vi "Go.vi"(8 "Timing Data (Go Down and Dispense)":T1(array[cluster]), 9 "Timing Values":dbl[](array[numeric]), 10 "Control In":T2={"I-O.lvclass"=refnum, "Motion.lvclass"=refnum, "Dispenser.lvclass"=refnum}, 11 "CAD Dispense in":refnum<class "CAD Dispense.lvclass">) -> (2 "Control Out":T2, 3 "CAD Dispense Out":refnum<class "CAD Dispense.lvclass">)   [LabVIEW 2016, in "CAD Dispense.lvclass"]
uses:
  CAD Dispense.lvclass
  Controller/Controllers.ctl
  Controller/I-O/I-O.lvclass
  Controller/Motion/A3200/A3200.lvclass
  Controller/Dispenser/Dispenser.lvclass
  Controller/Motion/Motion.lvclass
  CAD Dispense.lvclass/CAD Dispense.ctl
  Controller/Controller.lvclass
panel:
  out "Numeric":i32
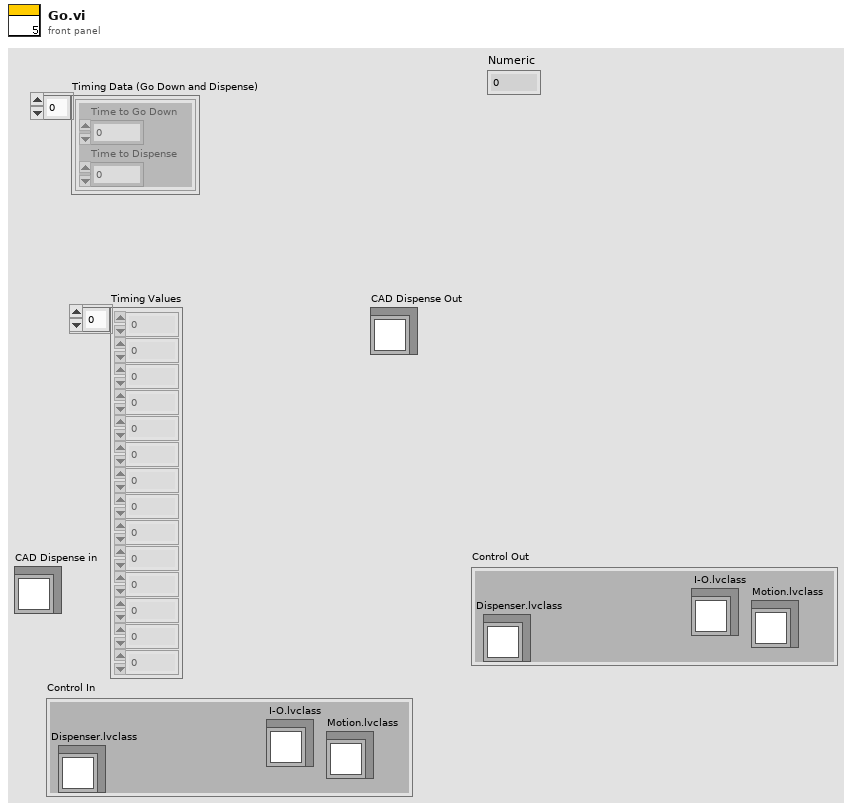
[diagram p1: front panel]
types:
  T1 = cluster{"Time to Go Down":dbl, "Time to Dispense":dbl}[]
  T2 = typedef "Controller.lvclass/Controllers.ctl" = cluster{"I-O.lvclass":refnum<class "I-O.lvclass">, "Motion.lvclass":refnum<class "Motion.lvclass">, "Dispenser.lvclass":refnum<class "Dispenser.lvclass">}
  T3 = cluster{"Motion":dbl[][], "Center":dbl[], "Circle?":bool, "CW/CCW":dbl}[]
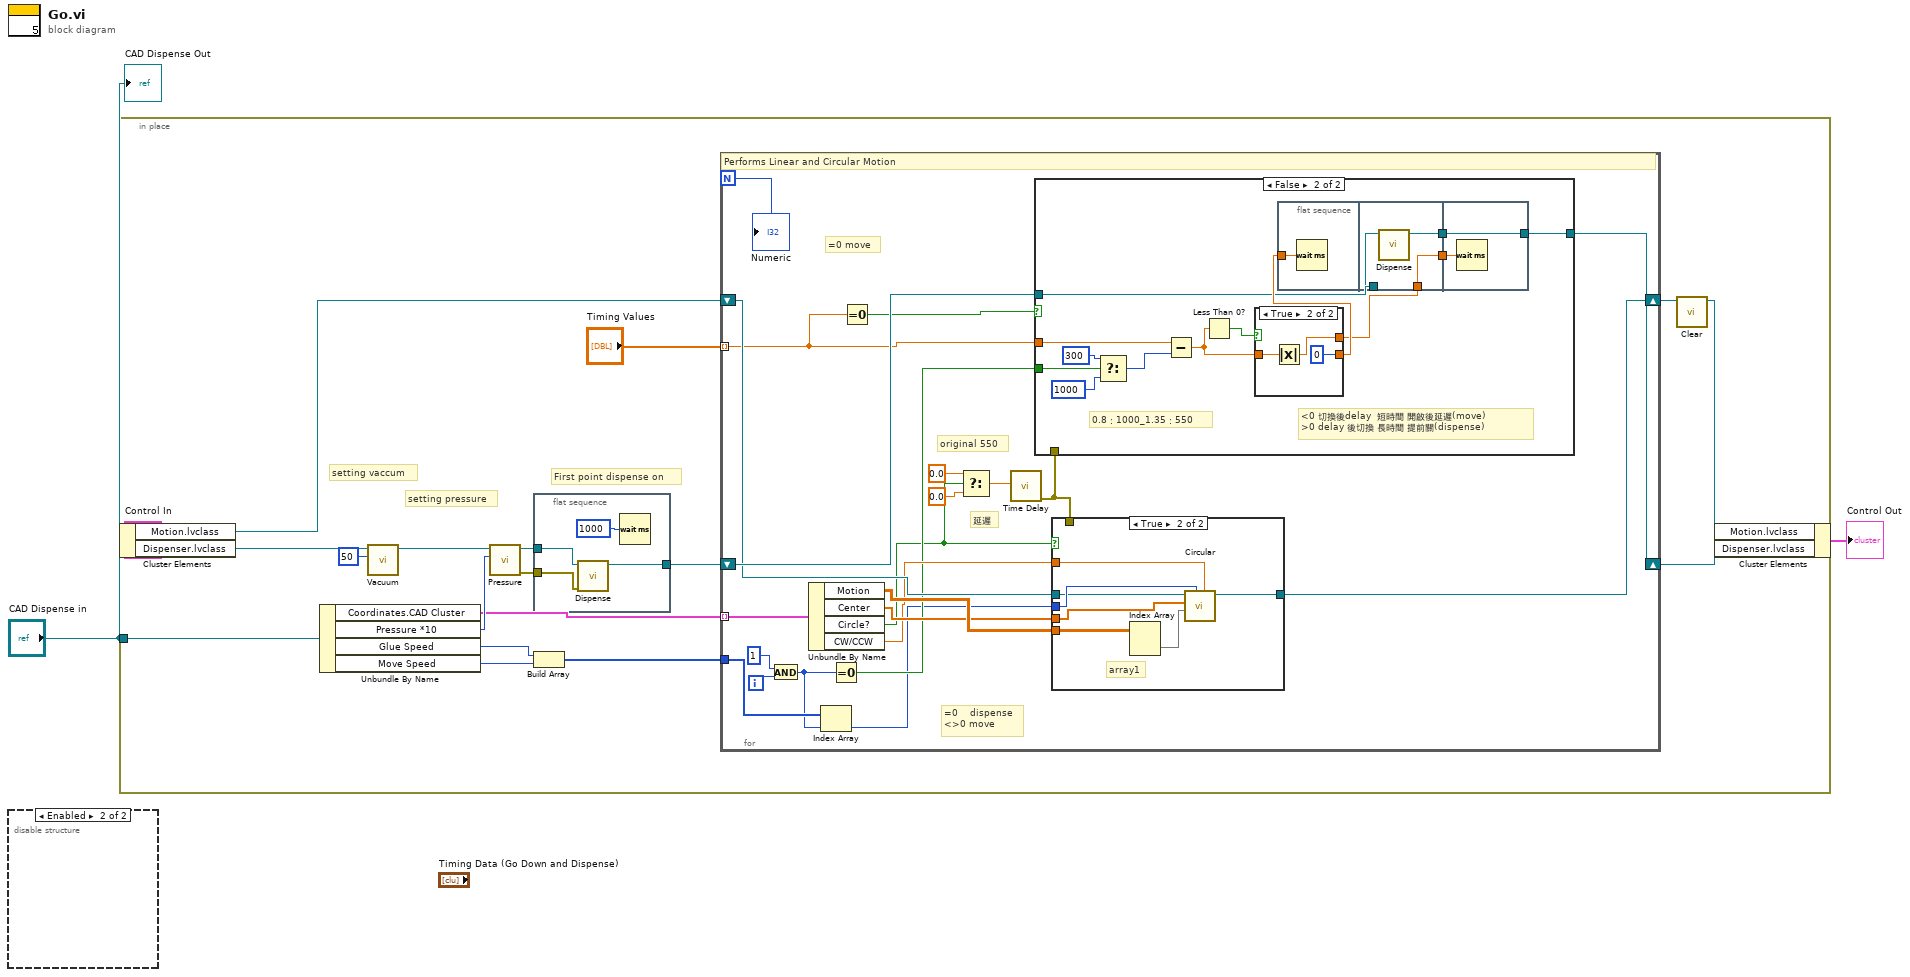
[diagram p0: block diagram]
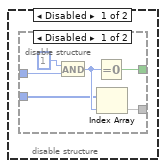
[diagram p2: hidden frame]
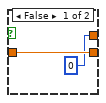
[diagram p5: hidden frame]
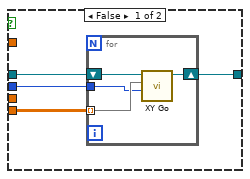
[diagram p6: hidden frame]
diagram:
  n1 = disable-structure shown="Enabled" {
    frame Disabled {
      n2 = disable-structure shown="Disabled" {
        disable-tunnel: [w8 _] -> _
        disable-tunnel: _ -> [w7 _]
        disable-tunnel: [w5 _] -> _
        disable-tunnel: _ -> [w4 _]
        frame Disabled {
          n3 = And(x=1, y=w7) -> (x .and. y?=w6:i32)
          n4 = Equal To 0?(x=w6) -> (x = 0?=w5:bool)
          n5 = Index Array(array=w4, index=w6) -> (element=w8)
        }
        frame Enabled {
        }
      }
    }
    frame Enabled {
    }
  }
  n6 = in-place {
    in-place-border: "CAD Dispense in" -> [w25]
    # "setting pressure"
    # "setting vaccum"
    # "First point dispense on"
    n7 = in-place-cluster #1("Control In") -> ("Motion.lvclass"=w19:refnum<class "Motion.lvclass">, "Dispenser.lvclass"=w12:refnum<class "Dispenser.lvclass">)
    n8 = Unbundle By Name(w25) -> ("Coordinates.CAD Cluster"=w13:T3, "Pressure *10"=w16:i64, "Glue Speed"=w23:i32, "Move Speed"=w22:i32)
    n9 = call-dynamic "Vacuum.vi"("Vacuum Setting (0000)"=i64 50, "Dispenser in"=w12) -> ("Dispenser out"=w11:refnum<class "Dispenser.lvclass">)  [unwired: 8 in, 1 out]
    n10 = call-dynamic "Pressure.vi"("Pressure"=w16, "Dispenser in"=w11) -> ("error out"=w15:errorcluster, "Dispenser out"=w14:refnum<class "Dispenser.lvclass">)  [unwired: 8 in]
    n11 = flat-sequence {
      tunnel: [w28] -> w24
      tunnel: w15 -> [w27]
      tunnel: w14 -> [w29]
      frame #0 {
        n12 = call-dynamic "Dispense.vi"("error in (no error)"=w27, "Dispenser in"=w29) -> ("Dispenser out"=w28:refnum<class "Dispenser.lvclass">)  [unwired: 8 in, 1 out]
        n13 = Wait (ms)(milliseconds to wait=u32 1000) -> ()  [unwired: 1 out]
      }
    }
    n14 = Build Array(w23, w22) -> (w21:i32[])
    n15 = for {
      N -> [w31]
      tunnel: w13 -> [w51] mode=indexing
      tunnel: "Timing Values" -> [w38] mode=indexing
      tunnel: w21 -> [w44]
      shift-right: [w46] -> w26
      shift-left: w24 -> [w52]
      shift-right: [w45] -> w18
      shift-left: w19 -> [w48]
      i -> [w43]
      # "=0 move"
      # "=0    dispense\n<>0 move"
      # "延遲"
      # "original 550"
      # "Performs Linear and Circular Motion"
      n16 = And(x=1, y=w43) -> (x .and. y?=w41:i32)
      n17 = Unbundle By Name(w51) -> ("Motion"=w50:dbl[][], "Center"=w49:dbl[], "Circle?"=w36:bool, "CW/CCW"=w47:dbl)
      n18 = Index Array(array=w44, index=w41) -> (element=w39:i32)
      n19 = Equal To 0?(x=w41) -> (x = 0?=w40:bool)
      n20 = Equal To 0?(x=w38) -> (x = 0?=w37:bool)
      n21 = Select(t=0.0, s=w36, f=0.0) -> (s? t:f=w33:dbl)
      n22 = call "Time Delay"("Delay Time (s)"=w33) -> ("error out"=w32:errorcluster)  [unwired: 10 in]
      n23 = case shown="False" w37 {
        tunnel: w52 -> [w53 w61]
        tunnel: w38 -> [_ w58]
        tunnel: [w53 w57] -> w46
        tunnel: w40 -> [_ w56]
        tunnel: w32 -> [_ _]
        frame True {
        }
        frame False {
          # "<0 切換後delay  短時間 開啟後延遲(move)\n>0 delay 後切換 長時間 提前關(dispense)"
          # "0.8：1000_1.35：550"
          n24 = Select(t=300, s=w56, f=1000) -> (s? t:f=w60:i32)
          n25 = Subtract(x=w58, y=w60) -> (x-y=w59:dbl)
          n26 = Less Than 0?(x=w59) -> (x < 0?=w64:bool)
          n27 = case shown="True" w64 {
            tunnel: [w74 u32 0 ("milliseconds to wait")] -> w63
            tunnel: w59 -> [w74 w77]
            tunnel: [u32 0 ("milliseconds to wait") w76] -> w62
            frame False {
            }
            frame True {
              n28 = Absolute Value(x=w77) -> (abs(x)=w76:dbl)
            }
          }
          n29 = flat-sequence {
            tunnel: w63 -> [w67]
            tunnel: w61 -> [w69]
            tunnel: [w70] -> w66
            tunnel: w62 -> [w70]
            tunnel: [w68] -> w65
            tunnel: w66 -> [w72]
            tunnel: w65 -> [w71]
            tunnel: [w71] -> w57
            frame #0 {
              n30 = Wait (ms)(milliseconds to wait=w67) -> ()  [unwired: 1 out]
            }
            frame #1 {
              n31 = call-dynamic "Dispense.vi"("Dispenser in"=w69) -> ("Dispenser out"=w68:refnum<class "Dispenser.lvclass">)  [unwired: 9 in, 1 out]
            }
            frame #2 {
              n32 = Wait (ms)(milliseconds to wait=w72) -> ()  [unwired: 1 out]
            }
          }
        }
      }
      n33 = case shown="True" w36 {
        tunnel: [w78 w86] -> w45
        tunnel: w47 -> [_ w89]
        tunnel: w50 -> [w80 w92]
        tunnel: w49 -> [_ w91]
        tunnel: w48 -> [w81 w87]
        tunnel: w39 -> [w79 w88]
        tunnel: w32 -> [_ _]
        frame False {
          n34 = for {
            tunnel: w80 -> [w84] mode=indexing
            shift-right: [w85] -> w78
            shift-left: w81 -> [w82]
            tunnel: w79 -> [w83]
            n35 = call-dynamic "XY Go.vi"("Speed"=w83, "XY"=w84, "Motion in"=w82) -> ("Motion out"=w85:refnum<class "Motion.lvclass">)  [unwired: 7 in, 1 out]
          }
        }
        frame True {
          # "array1"
          n36 = Index Array(array=w92) -> (element=w90:dbl[])  [unwired: 2 in]
          n37 = call-dynamic "Circular.vi"("Direction"=w89, "Speed"=w88, "XY End"=w90, "XY Center"=w91, "Motion in"=w87) -> ("Motion out"=w86:refnum<class "Motion.lvclass">)  [unwired: 5 in, 1 out]
        }
      }
      "Numeric" <- w31
    }
    n38 = call "Clear.vi"("Motion in"=w18) -> ("Motion out"=w17:refnum<class "Motion.lvclass">)  [unwired: 9 in, 1 out]
    n39 = in-place-cluster #1("Motion.lvclass"=w17, "Dispenser.lvclass"=w26) -> (→"Control Out":T2)
  }
  "CAD Dispense Out" <- "CAD Dispense in"
